vi "9-v1-v2.vi"(3 "this":i32, 4 "button":i32, 5 "shift in":bool) -> (0 "next state":i32, 1 "shift out":bool)   [LabVIEW 2017]
panel:
  out "settings out":T1
  in  "settings in":T1={"Auto1"=TRUE, "Auto2"=TRUE, "Rel1"=TRUE, "Rel2"=TRUE, "Filt1"=TRUE, "Filt2"=TRUE, "Rate"=enum."Slow", "Range1"=enum."10mV", "Range2"=enum."100mV", "Filt3"=TRUE, "Filt4"=TRUE, "Rel temp 1"=TRUE, "Analog1"=FALSE, "Analog2"=FALSE, "Analog temp 1"=FALSE, "Digital1"=TRUE, "Digital2"=TRUE, "Digital temp 1 "=TRUE, "Window1"=enum."0,01%", "Window2"=enum."0,01%", "Window temp 1"=enum."0,01%", "RDGS1"="010", "RDGS2"="010", "RDGS temp 1"="010", "Type_type1"=TRUE, "Type_type2"=TRUE, "Type_type temp 1"=TRUE, "LSync"=FALSE, "Unit"=enum."C", "Sens"=TRUE, "Type tcoupl"=enum."J", "Junc"=TRUE, "prevState"=0, "Rel temp 2"=TRUE, "Analog temp 2"=FALSE, "Digital temp 2"=TRUE, "Type_type temp 2"=TRUE, "RDGS temp 2"="010", "Window temp 2"=enum."0,01%"}
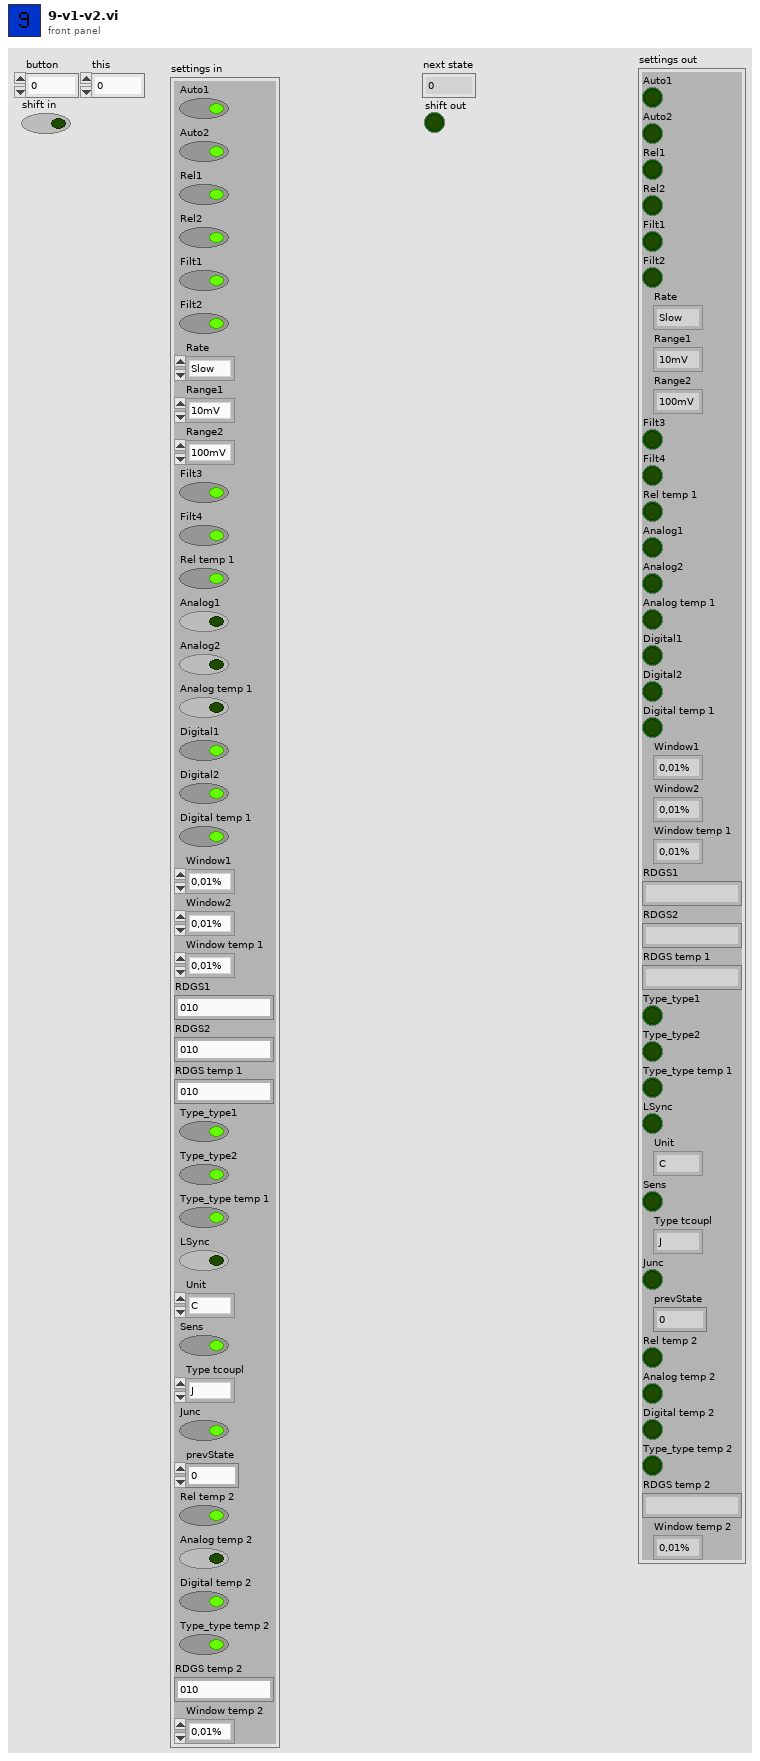
[diagram p1: front panel]
types:
  T1 = cluster{"Auto1":bool, "Auto2":bool, "Rel1":bool, "Rel2":bool, "Filt1":bool, "Filt2":bool, "Rate":enum16{"Slow", "Med", "Fast"}, "Range1":enum16{"10mV", "100mV", "1V", "10V", "100V"}, "Range2":enum16{"100mV", "1V", "10V"}, "Filt3":bool, "Filt4":bool, "Rel temp 1":bool, "Analog1":bool, "Analog2":bool, "Analog temp 1":bool, "Digital1":bool, "Digital2":bool, "Digital temp 1 ":bool, "Window1":enum16{"0,01%", "0,1%", "1%", "10%", "None"}, "Window2":enum16{"0,01%", "0,1%", "1%", "10%", "None"}, "Window temp 1":enum16{"0,01%", "0,1%", "1%", "10%", "None"}, "RDGS1":string, "RDGS2":string, "RDGS temp 1":string, "Type_type1":bool, "Type_type2":bool, "Type_type temp 1":bool, "LSync":bool, "Unit":enum16{"C", "K", "F"}, "Sens":bool, "Type tcoupl":enum16{"J", "K", "T", "E", "R", "S", "B", "N"}, "Junc":bool, "prevState":i32, "Rel temp 2":bool, "Analog temp 2":bool, "Digital temp 2":bool, "Type_type temp 2":bool, "RDGS temp 2":string, "Window temp 2":enum16{"0,01%", "0,1%", "1%", "10%", "None"}}
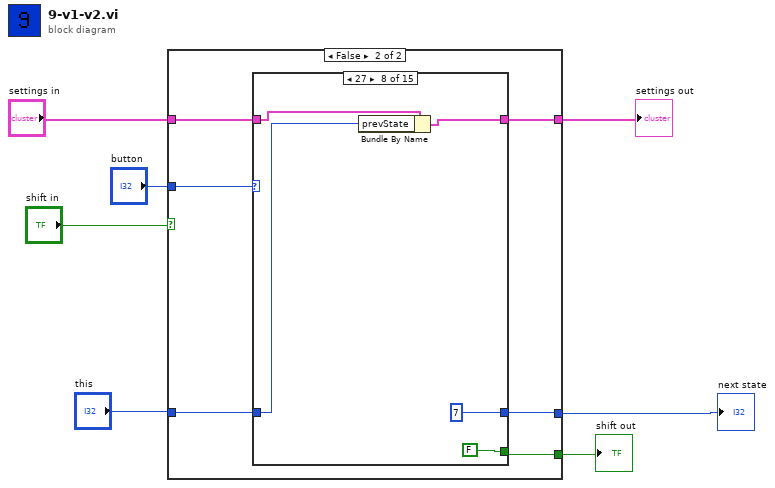
[diagram p0: block diagram]
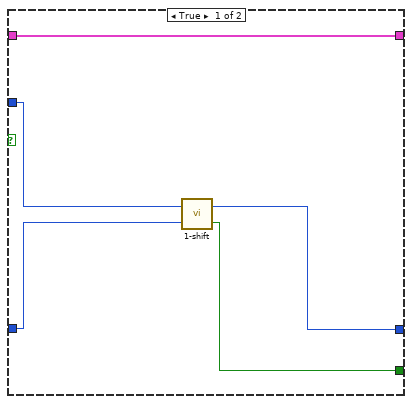
[diagram p2: hidden frame]
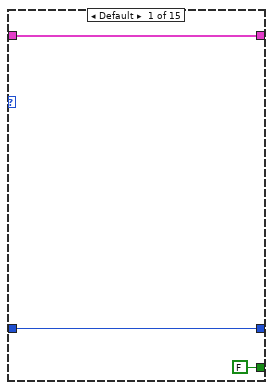
[diagram p3: hidden frame]
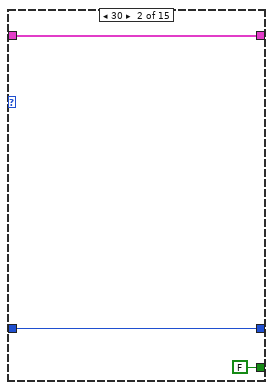
[diagram p4: hidden frame]
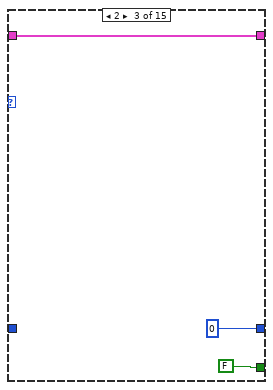
[diagram p5: hidden frame]
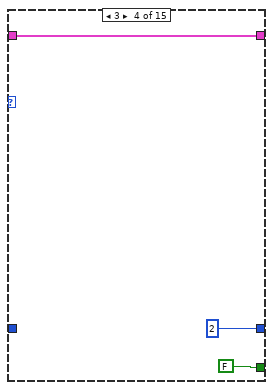
[diagram p6: hidden frame]
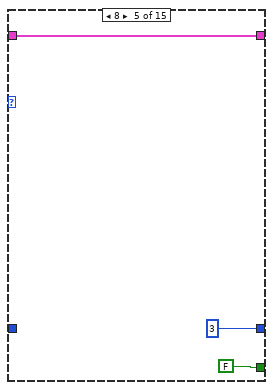
[diagram p7: hidden frame]
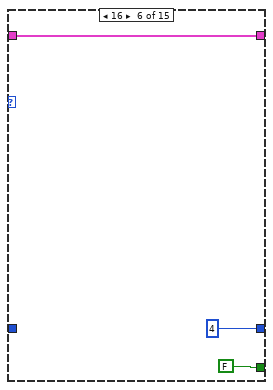
[diagram p8: hidden frame]
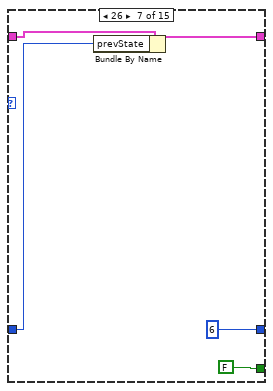
[diagram p9: hidden frame]
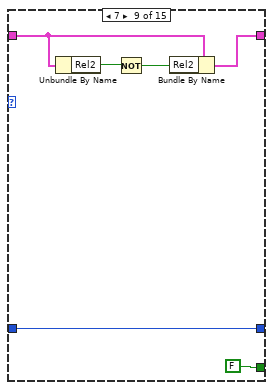
[diagram p10: hidden frame]
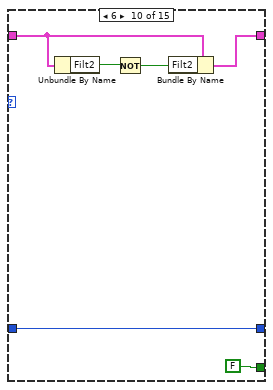
[diagram p11: hidden frame]
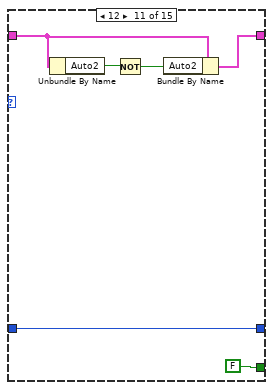
[diagram p12: hidden frame]
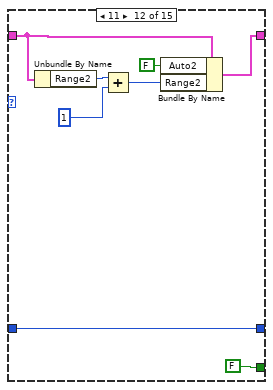
[diagram p13: hidden frame]
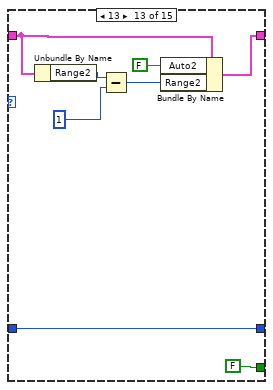
[diagram p14: hidden frame]
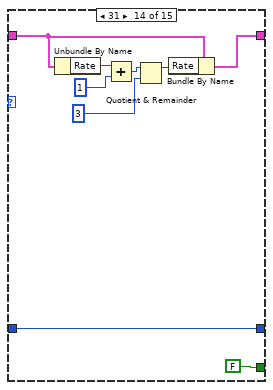
[diagram p15: hidden frame]
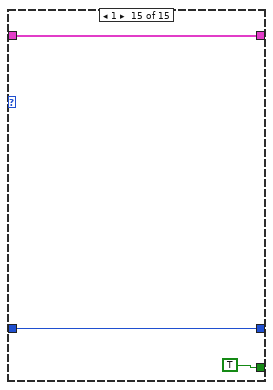
[diagram p16: hidden frame]
diagram:
  n1 = case shown="False" "shift in" {
    tunnel: "button" -> [w12 w18]
    tunnel: [w11 w17] -> w5
    tunnel: "this" -> [w10 w16]
    tunnel: [w8 w15] -> w3
    tunnel: "settings in" -> [w9 w14]
    tunnel: [w9 w13] -> w2
    frame True {
      n2 = call "1-shift.vi"("this"=w10, "button"=w12) -> ("shift"=w8:bool, "next state"=w11:i32)
    }
    frame False {
      n3 = case shown="27" w18 {
        tunnel: [w20 w23 0 2 3 4 6 7 w51 w57 w63 w71 w79 w88 w92] -> w17
        tunnel: w16 -> [w20 w23 _ _ _ _ w37 w42 w51 w57 w63 w71 w79 w88 w92]
        tunnel: [FALSE ("shift") FALSE ("shift") FALSE ("shift") FALSE ("shift") FALSE ("shift") FALSE ("shift") FALSE ("shift") FALSE ("shift") FALSE ("shift") FALSE ("shift") FALSE ("shift") FALSE ("shift") FALSE ("shift") FALSE ("shift") TRUE ("shift")] -> w15
        tunnel: w14 -> [w21 w24 w25 w28 w31 w34 w39 w44 w48 w54 w60 w67 w75 w87 w90]
        tunnel: [w21 w24 w25 w28 w31 w34 w38 w43 w47 w53 w59 w70 w78 w86 w90] -> w13
        frame Default {
        }
        frame 30 {
        }
        frame 2 {
        }
        frame 3 {
        }
        frame 8 {
        }
        frame 16 {
        }
        frame 26 {
          n4 = Bundle By Name(cluster=w39, "prevState"=w37) -> (w38:T1)
        }
        frame 27 {
          n5 = Bundle By Name(cluster=w44, "prevState"=w42) -> (w43:T1)
        }
        frame 7 {
          n6 = Unbundle By Name(w48) -> ("Rel2"=w50:bool)
          n7 = Not(x=w50) -> (.not. x?=w49:bool)
          n8 = Bundle By Name(cluster=w48, "Rel2"=w49) -> (w47:T1)
        }
        frame 6 {
          n9 = Unbundle By Name(w54) -> ("Filt2"=w56:bool)
          n10 = Not(x=w56) -> (.not. x?=w55:bool)
          n11 = Bundle By Name(cluster=w54, "Filt2"=w55) -> (w53:T1)
        }
        frame 12 {
          n12 = Unbundle By Name(w60) -> ("Auto2"=w62:bool)
          n13 = Not(x=w62) -> (.not. x?=w61:bool)
          n14 = Bundle By Name(cluster=w60, "Auto2"=w61) -> (w59:T1)
        }
        frame 11 {
          n15 = Unbundle By Name(w67) -> ("Range2"=w66:enum16{"100mV", "1V", "10V"})
          n16 = Add(x=w66, y=1) -> (x+y=w68:i32)
          n17 = Bundle By Name(cluster=w67, "Auto2"=FALSE ("Auto1"), "Range2"=w68) -> (w70:T1)
        }
        frame 13 {
          n18 = Unbundle By Name(w75) -> ("Range2"=w74:enum16{"100mV", "1V", "10V"})
          n19 = Subtract(x=w74, y=1) -> (x-y=w76:i32)
          n20 = Bundle By Name(cluster=w75, "Auto2"=FALSE ("Auto1"), "Range2"=w76) -> (w78:T1)
        }
        frame 31 {
          n21 = Unbundle By Name(w87) -> ("Rate"=w85:enum16{"Slow", "Med", "Fast"})
          n22 = Add(x=w85, y=1) -> (x+y=w83:i32)
          n23 = Quotient & Remainder(x=w83, y=3) -> (x-y*floor(x/y)=w82:i32)  [unwired: 1 out]
          n24 = Bundle By Name(cluster=w87, "Rate"=w82) -> (w86:T1)
        }
        frame 1 {
        }
      }
    }
  }
  "next state" <- w5
  "shift out" <- w3
  "settings out" <- w2
